vi "TANGO Control.vi"() -> ()   [LabVIEW 2013]
uses:
  <userlib>/Tango_DLL/Tango_DLL.lvlib
panel:
  in  "stop":bool
  out "error out 2":errorcluster
  out "Pos":dbl[](array[numeric])
  in  "error in (no error) 2":errorcluster
  out "error out":errorcluster
  in  "TANGO VISA Port":refnum<visa-resource-name>
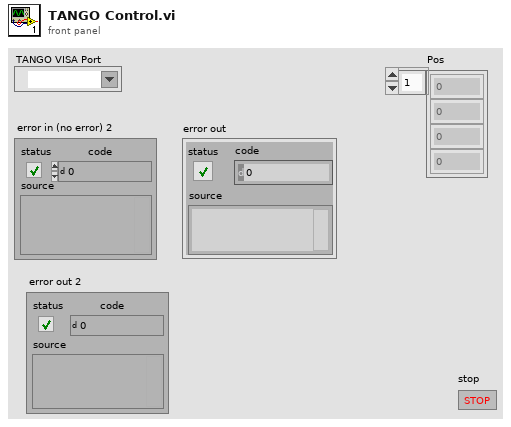
[diagram p1: front panel]
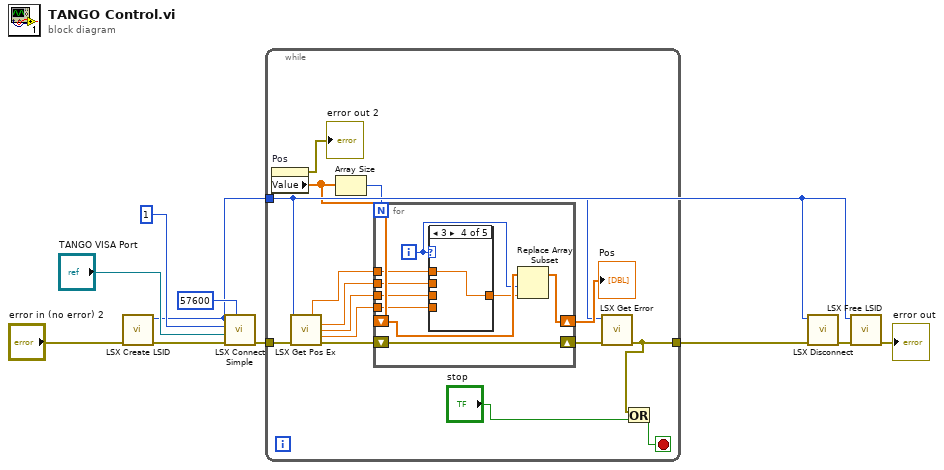
[diagram p0: block diagram]
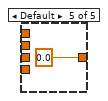
[diagram p5: hidden frame]
diagram:
  n1 = call <userlib>:"LSX Create LSID.vi"("error in (no error)"="error in (no error) 2") -> ("error out"=w10:errorcluster, "plLSID out"=w1:i32)  [unwired: 8 in, 1 out]
  n2 = call <userlib>:"LSX Connect Simple.vi"("lABaudRate"=57600, "error in (no error)"=w10, "pcAComName"="TANGO VISA Port", "lAnInterfaceType"=1, "lLSID"=w1) -> ("error out"=w2:errorcluster)  [unwired: 4 in, 2 out]
  n3 = while {
    tunnel: [w12] -> w3
    tunnel: w2 -> [w20]
    tunnel: w1 -> [w14]
    stop <- w13 stop-if-true
    n4 = property on="Pos" class="Arr (strict)"() -> (error out=→"error out 2":errorcluster, "Value"=w22:dbl[])  [unwired: 2 in, 1 out]
    n5 = call <userlib>:"LSX Get Pos Ex.vi"("lLSID"=w14, "error in (no error)"=w20) -> ("pdR out"=w15:dbl, "pdX out"=w16:dbl, "pdY out"=w17:dbl, "pdZ out"=w18:dbl, "error out"=w19:errorcluster)  [unwired: 8 in, 1 out]
    n6 = Array Size(array=w22) -> (size(s)=w25:i32)
    n7 = for {
      N: w25 -> [_]
      tunnel: w16 -> [w33]
      tunnel: w17 -> [w32]
      tunnel: w18 -> [w31]
      tunnel: w15 -> [w30]
      shift-right: [w27] -> w23
      shift-left: w22 -> [w34]
      shift-right: [w26] -> w24
      shift-left: w19 -> [w26]
      i -> [w29]
      n8 = case shown="3" w29 {
        tunnel: w33 -> [w35 _ _ _ _]
        tunnel: w32 -> [_ w36 _ _ _]
        tunnel: w31 -> [_ _ w37 _ _]
        tunnel: w30 -> [_ _ _ w38 _]
        tunnel: [w35 w36 w37 w38 0.0 ("pdA out")] -> w28
        frame 0 {
        }
        frame 1 {
        }
        frame 2 {
        }
        frame 3 {
        }
        frame Default {
        }
      }
      n9 = Replace Array Subset(array=w34, new element=w28, index=w29) -> (w27:dbl[])
    }
    "Pos" <- w23
    n10 = call <userlib>:"LSX Get Error.vi"("error in (no error)"=w24, "lLSID"=w14) -> ("error out"=w12:errorcluster)  [unwired: 7 in, 2 out]
    n11 = Or(x=w12, y="stop") -> (x .or. y?=w13:bool)
  }
  n12 = call <userlib>:"LSX Disconnect.vi"("error in (no error)"=w3, "lLSID"=w1) -> ("error out"=w5:errorcluster)  [unwired: 8 in, 1 out]
  n13 = call <userlib>:"LSX Free LSID.vi"("error in (no error)"=w5, "lLSID"=w1) -> ("error out"=→"error out":errorcluster)  [unwired: 8 in, 1 out]
